vi "Read Job.vi"(8 "error in (no error)":errorcluster, 11 "AIncome in":refnum<class "AIncome.lvclass">) -> (0 "error out":errorcluster, 2 "Job":string, 3 "AIncome out":refnum<class "AIncome.lvclass">)   [LabVIEW 2020, in "AIncome.lvclass"]
uses:
  AIncome.lvclass
  AIncome.lvclass/AIncome.ctl
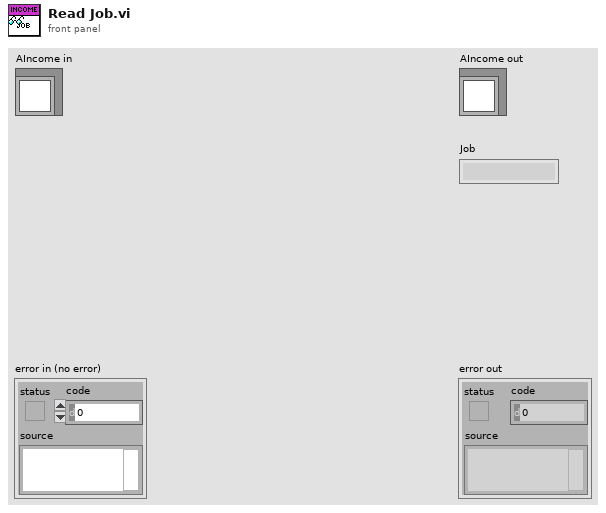
[diagram p1: front panel]
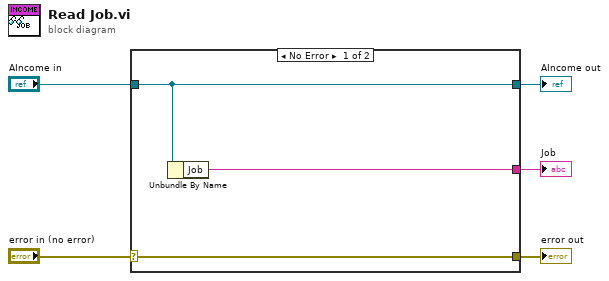
[diagram p0: block diagram]
diagram:
  n1 = case shown="No Error" "error in (no error)" {
    selector: "error in (no error)" -> [w8 w9]
    tunnel: [w8 w9] -> w4
    tunnel: [w7 w10] -> w2
    tunnel: "AIncome in" -> [w7 w10]
    tunnel: [w6 _] -> w1
    frame No Error {
      n2 = Unbundle By Name(w7) -> ("Job"=w6:string)
    }
    frame Error {
    }
  }
  "error out" <- w4
  "AIncome out" <- w2
  "Job" <- w1
